vi "hla_incoming_queue_instance_5.vi"(4 "timeout in ms (-1)":i32, 5 "error in (no error)":errorcluster) -> (16 "entity_array":T1[](array[typedef]), 17 "time_step":dbl, 18 "end_simulation":bool, 19 "error out":errorcluster)   [LabVIEW 2016]
uses:
  objects_and_interfaces/InteractionRoot.C2WInteractionRoot.FederateJoinInteraction.ctl
  utilities/runtime/support/controls/queue_assistant_actions.ctl
  utilities/runtime/support/controls/event_assistant_actions.ctl
  utilities/pre-build/support/base_components/controls/incoming_queue_action.ctl
panel:
  out "InteractionRoot.C2WInteractionRoot.FederateJoinInteraction":T1
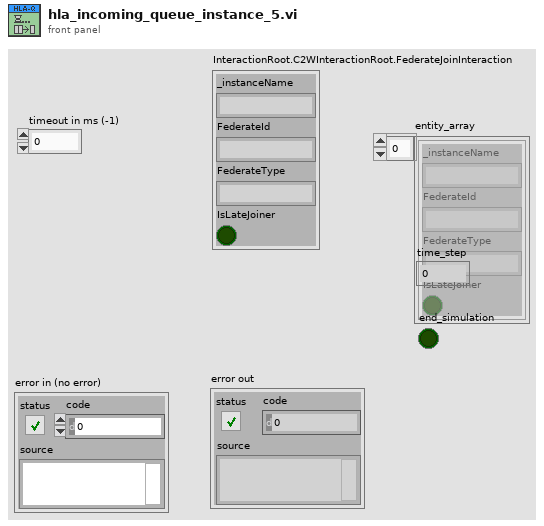
[diagram p1: front panel]
types:
  T1 = typedef "InteractionRoot.C2WInteractionRoot.FederateJoinInteraction.ctl" = cluster{"_instanceName":string, "FederateId":string, "FederateType":string, "IsLateJoiner":bool}
  T2 = typedef "incoming_queue_action.ctl" = enum16{"exit", "process_queue", "wait_on_action"}
  T3 = typedef "event_assistant_actions.ctl" = enum16{"--- unused ---", "destroy", "fire", "get_ref", "init"}
  T4 = typedef "queue_assistant_actions.ctl" = enum16{"--- unused ---", "bulk_enq_ahead", "bulk_enq_behind", "destroy", "empty?", "enq_ahead", "enq_behind", "flush", "get_queues", "init"}
  T5 = typedef "queue_references.ctl" = cluster{"entities_in":refnum<queue>, "entities_out":refnum<queue>, "timestep":refnum<queue>, "response":refnum<queue>}
  T6 = typedef "entity.ctl" = cluster{"type":T7, "classPath":string, "params":string[][], "instanceName":string}
  T7 = typedef "entity_type.ctl" = string
  T8 = typedef "user_events.ctl" = enum16{"abort", "do-step", "sim-end"}
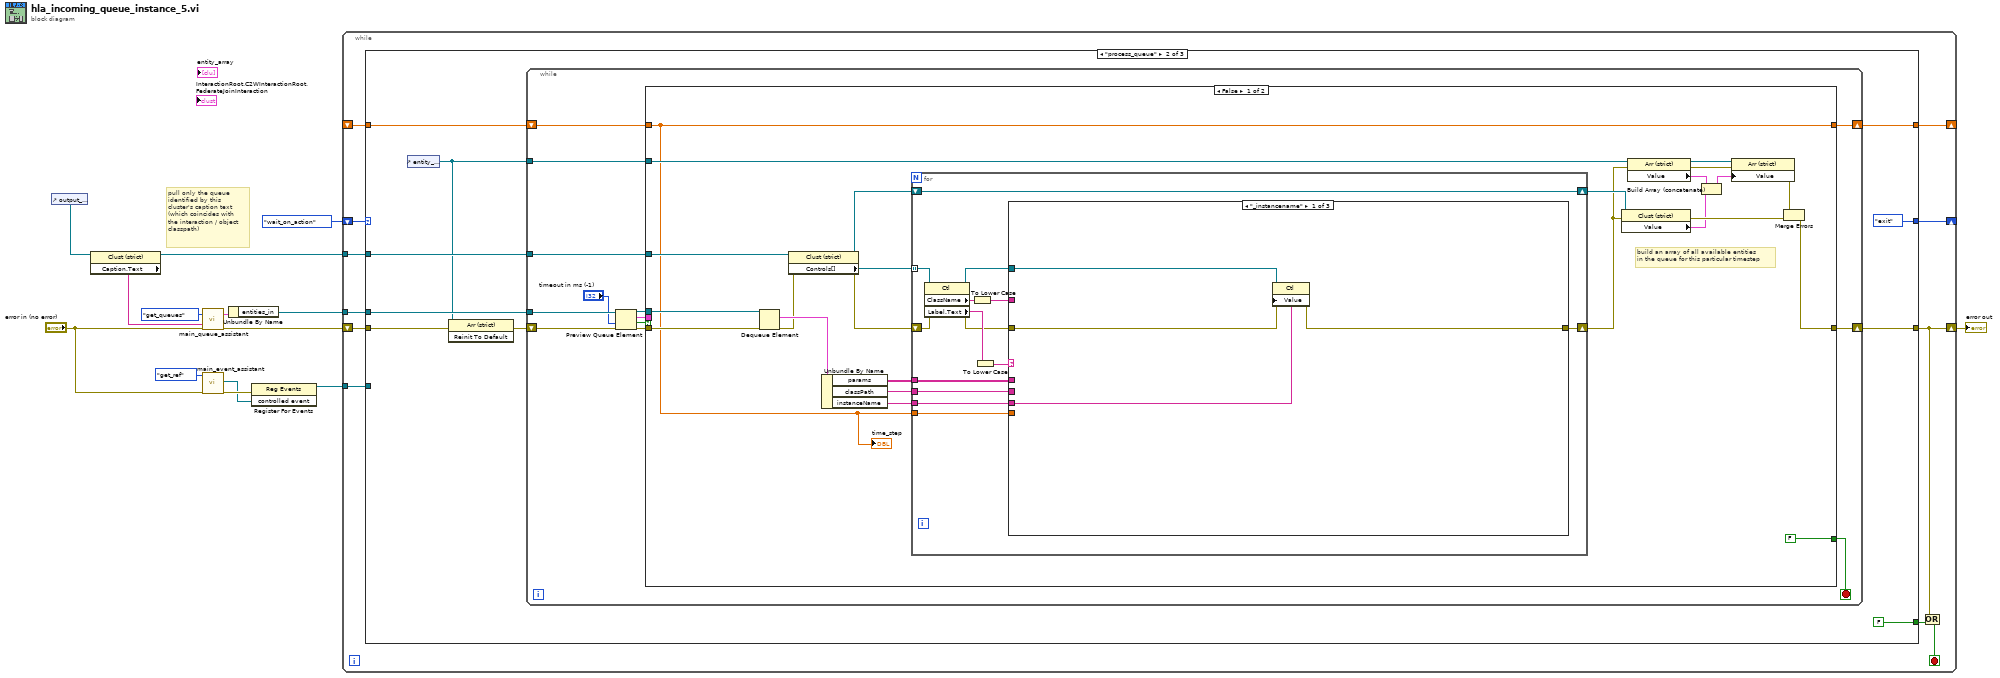
[diagram p0: block diagram]
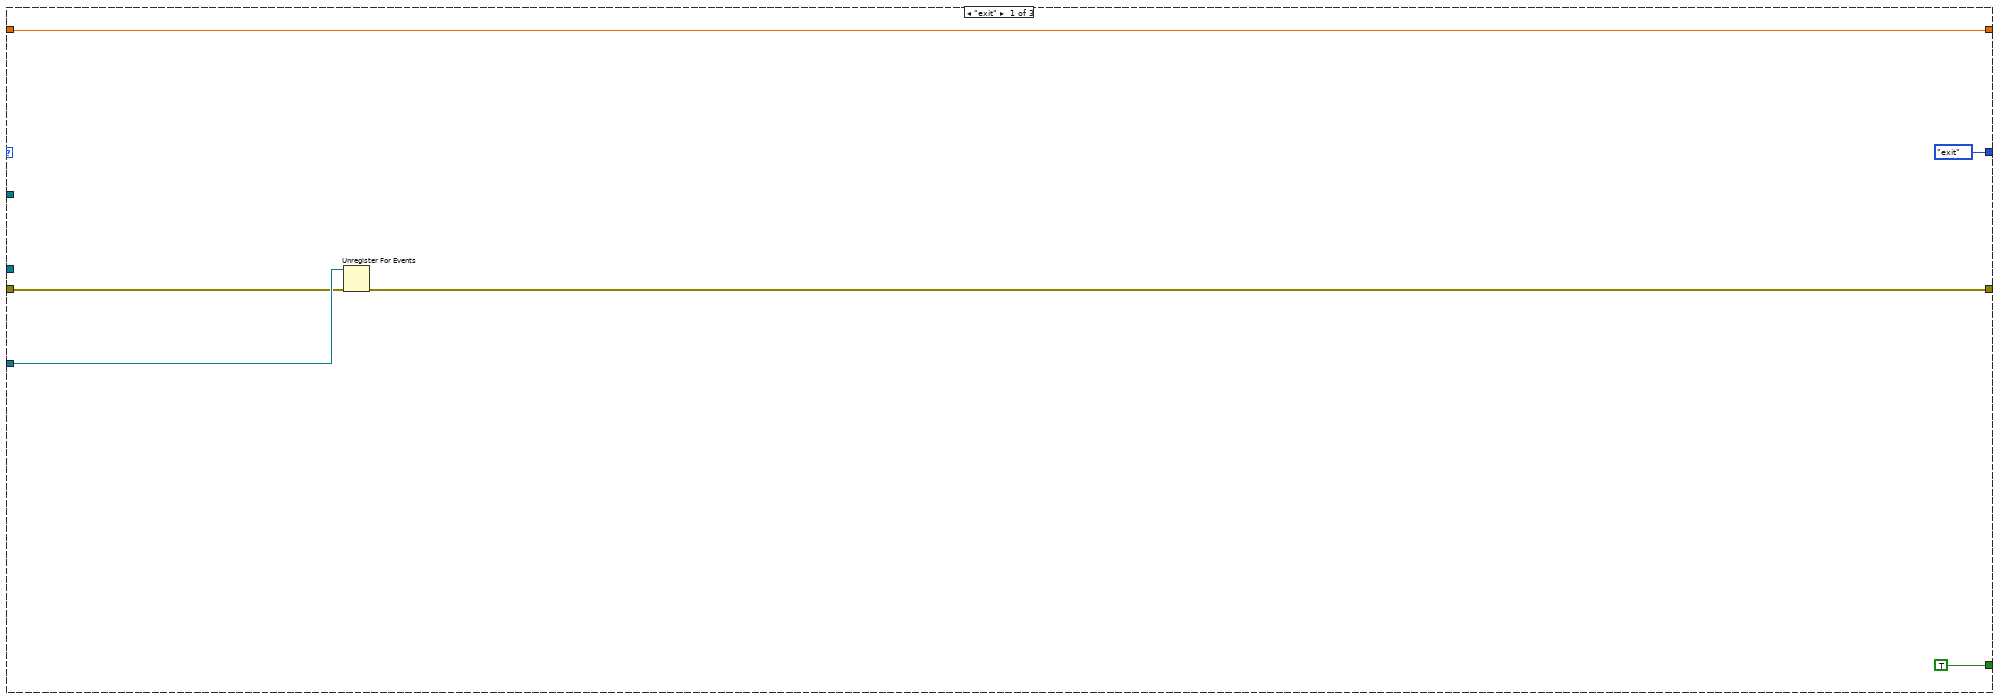
[diagram p2: hidden frame]
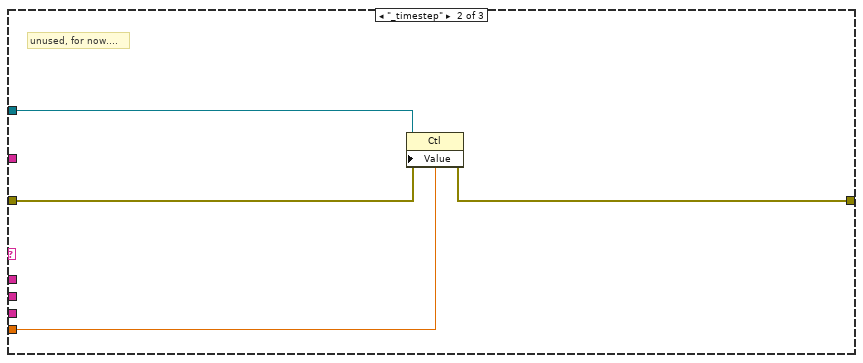
[diagram p3: hidden frame]
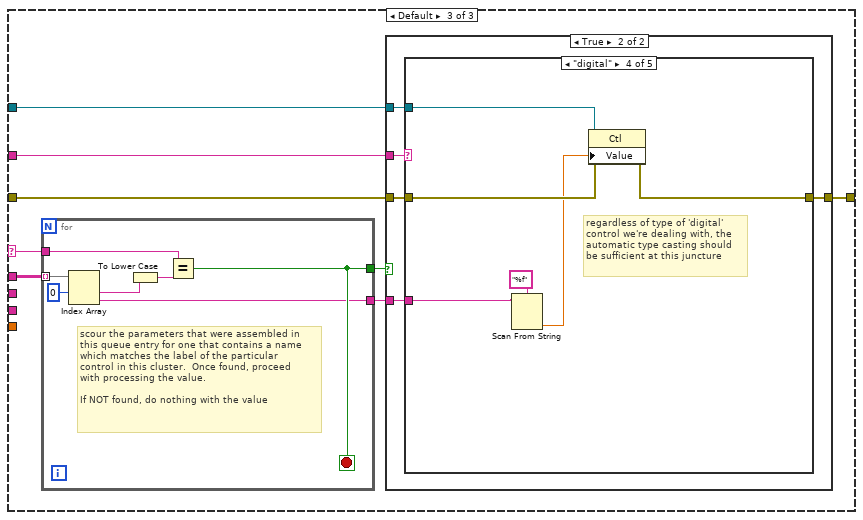
[diagram p4: hidden frame]
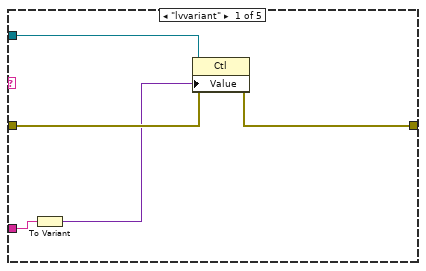
[diagram p6: hidden frame]
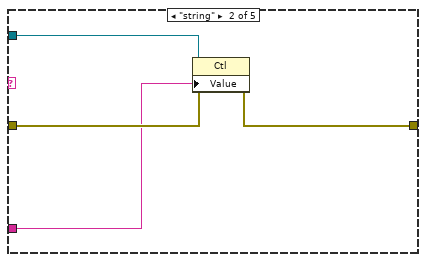
[diagram p7: hidden frame]
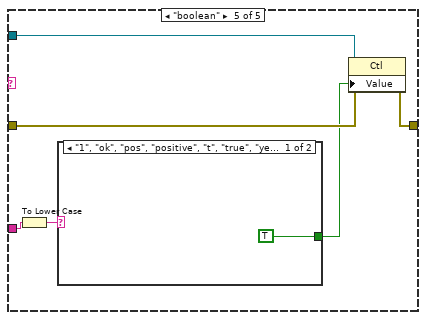
[diagram p9: hidden frame]
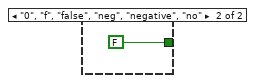
[diagram p10: hidden frame]
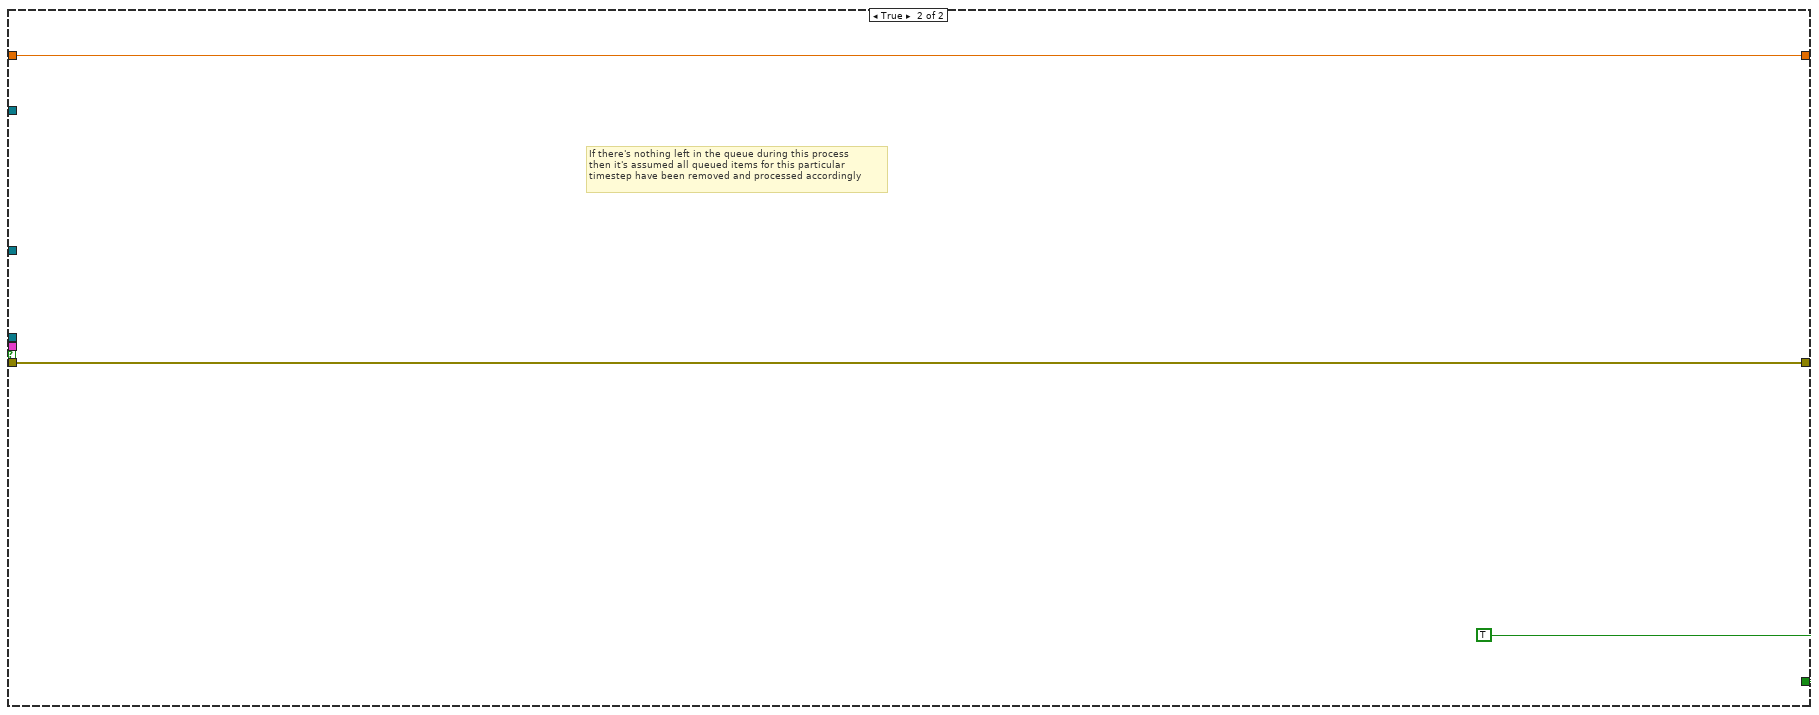
[diagram p11: hidden frame]
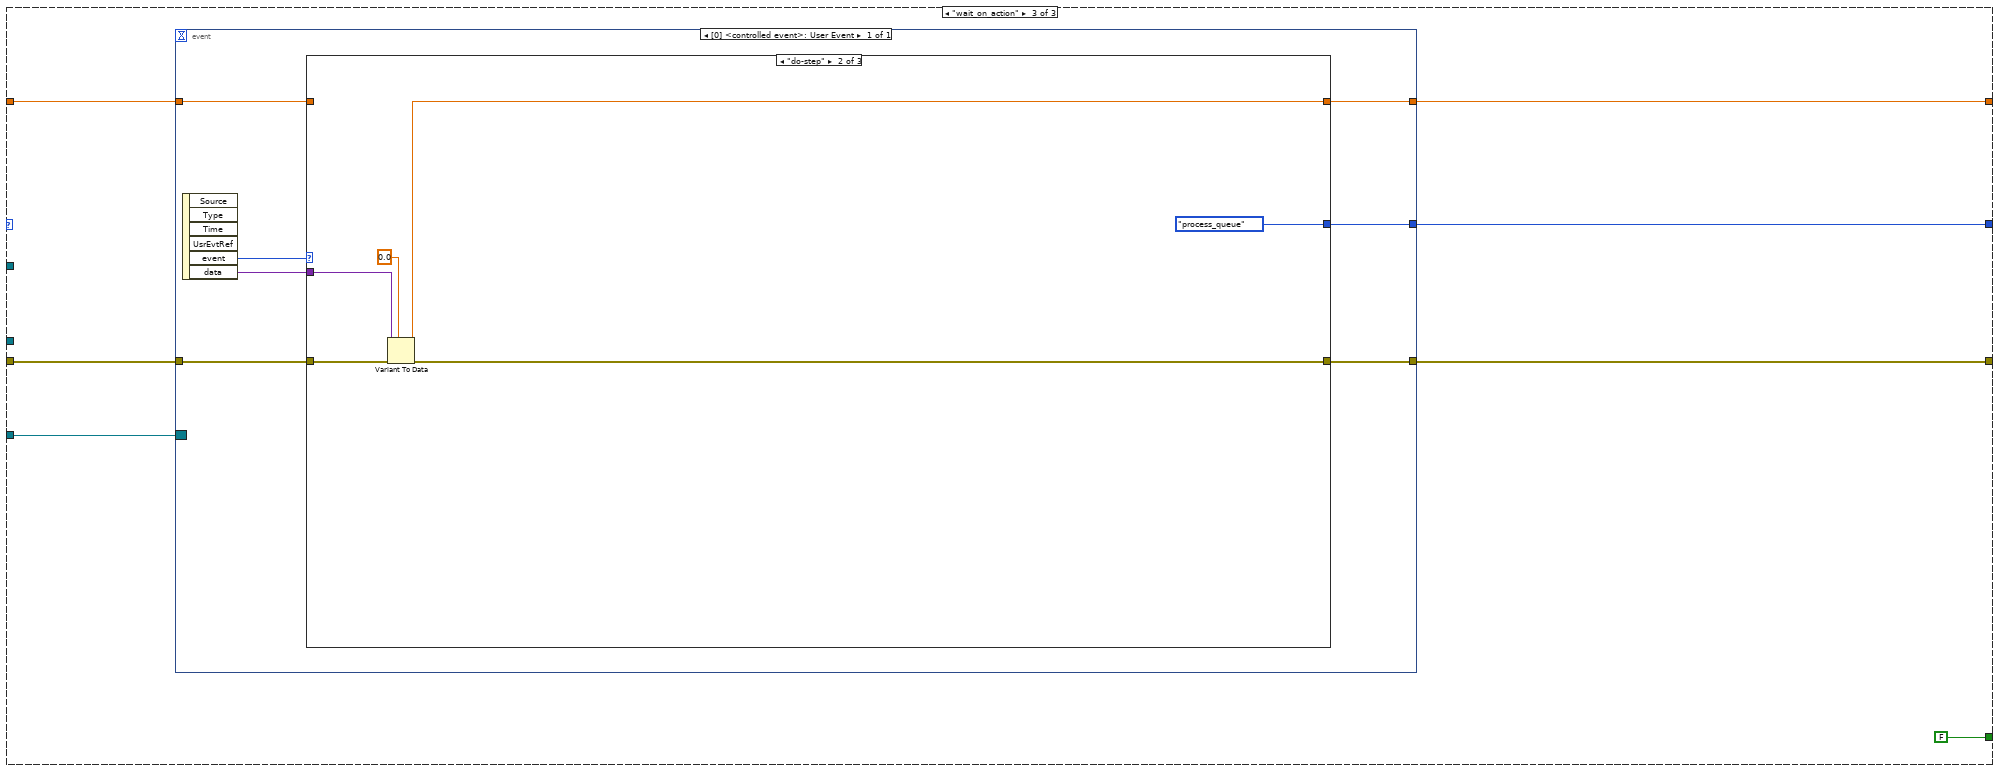
[diagram p12: hidden frame]
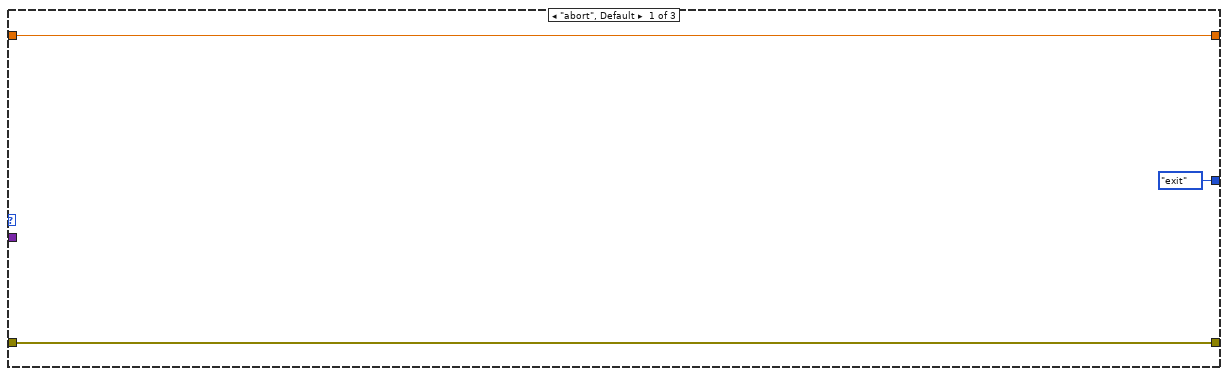
[diagram p13: hidden frame]
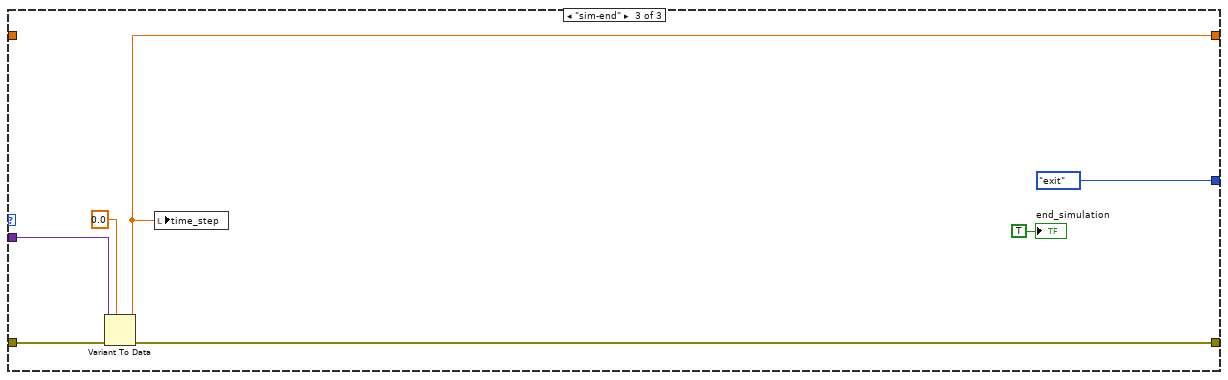
[diagram p14: hidden frame]
diagram:
  # "pull only the queue \nidentified by this \ncluster's caption text\n(which coincides with\nthe interaction / object\nclasspath)"
  n1 = control-ref of="output_cluster"() -> (w3:refnum<vi>)
  n2 = property class="Clust (strict)"(reference=w3) -> (reference out=w11:refnum<vi>, "Caption.Text"=w12:string)  [unwired: 1 in, 1 out]
  n3 = call "main_queue_assistant.vi"("action (enq_behind = def)"=queue_assistant_actions."get_queues" ("queue_action (enq_behind = def)"), "classpath / id (in)"=w12, "error in (no error)"="error in (no error)") -> ("refs (out)"=w2:T5, "error out"=w10:errorcluster)  [unwired: 14 in, 1 out]
  n4 = call "main_event_assistant.vi"("event_action (enq_behind = def)"=event_assistant_actions."get_ref", "error in (no error)"="error in (no error)") -> ("controlled event"=w6:refnum<user-event>, "error out"=w7:errorcluster)  [unwired: 16 in]
  n5 = Unbundle By Name(w2) -> ("entities_in"=w1:refnum<queue>)
  n6 = register-events(error in=w7, w6) -> (reference out=w4:refnum<event-registration>)  [unwired: 1 in, 1 out]
  n7 = while {
    tunnel: w1 -> [w25]
    tunnel: w11 -> [w24]
    shift-right: [w16] -> w13
    shift-left: w10 -> [w23]
    shift-right: [w19] -> _
    shift-left: incoming_queue_action."wait_on_action" -> [w22]
    tunnel: w4 -> [w21]
    shift-right: [w20] -> _
    shift-left: _ -> [w18]
    stop <- w15 stop-if-true
    n8 = case shown="\"process_queue\"" w22 {
      tunnel: w25 -> [_ w41 _]
      tunnel: [w26 w40 w152] -> w16
      tunnel: w24 -> [_ w39 _]
      tunnel: w23 -> [w27 w35 w154]
      tunnel: w21 -> [w28 _ w155]
      tunnel: [w31 w37 w153] -> w20
      tunnel: [incoming_queue_action."exit" incoming_queue_action."exit" w151] -> w19
      tunnel: w18 -> [w31 w36 w150]
      tunnel: [TRUE FALSE FALSE] -> w17
      frame "exit" {
        n9 = Unregister For Events(event registration refnum=w28, error in=w27) -> (error out=w26:errorcluster)
      }
      frame "process_queue" {
        n10 = control-ref of="entity_array"() -> (w33:refnum<vi>)
        n11 = invoke class="Arr (strict)" method="Reinit To Default"(reference=w33, error in=w35) -> (error out=w34:errorcluster)  [unwired: 1 in, 2 out]
        n12 = while {
          tunnel: w41 -> [w54]
          tunnel: w39 -> [w48]
          shift-right: [w49] -> w40
          shift-left: w34 -> [w47]
          shift-right: [w46] -> w37
          shift-left: w36 -> [w45]
          tunnel: w33 -> [w42]
          stop <- w43 stop-if-true
          n13 = Preview Queue Element(queue=w54, timeout in ms (-1)="timeout in ms (-1)", error in (no error)=w47) -> (queue out=w50:refnum<queue>, element=w44:T6, timed out?=w52:bool, error out=w51:errorcluster)
          n14 = case shown="False" w52 {
            tunnel: w51 -> [w75 w148]
            tunnel: w50 -> [w78 _]
            tunnel: [w77 w148] -> w49
            tunnel: w48 -> [w76 _]
            tunnel: w45 -> [w56 w147]
            tunnel: [w56 w147] -> w46
            tunnel: w44 -> [_ _]
            tunnel: [FALSE TRUE] -> w43
            tunnel: w42 -> [w74 _]
            frame False {
              # "build an array of all available entities\nin the queue for this particular timestep"
              n15 = Dequeue Element(queue=w78, error in (no error)=w75) -> (element=w72:T6, error out=w71:errorcluster)  [unwired: 1 in, 2 out]
              n16 = property class="Clust (strict)"(reference=w76, error in=w71) -> (reference out=w62:refnum<vi>, error out=w69:errorcluster, "Controls[]"=w70:refnum<vi>[])
              n17 = Unbundle By Name(w72) -> ("params"=w68:string[][], "classPath"=w67:string, "instanceName"=w55:string)
              n18 = for {
                tunnel: w70 -> [w91] mode=indexing
                tunnel: w68 -> [w87]
                shift-right: [w84] -> w58
                shift-left: w69 -> [w92]
                tunnel: w67 -> [w82]
                shift-right: [w81] -> w61
                shift-left: w62 -> [w81]
                tunnel: w56 -> [w80]
                tunnel: w55 -> [w79]
                n19 = property class="Ctl"(reference=w91, error in=w92) -> (reference out=w89:refnum<vi>, error out=w85:errorcluster, "ClassName"=w90:string, "Label.Text"=w86:string)
                n20 = To Lower Case(string=w90) -> (all lower case string=w88:string)
                n21 = To Lower Case(string=w86) -> (all lower case string=w83:string)
                n22 = case shown="\"_instancename\"" w83 {
                  selector: w83 -> [_ _ w101]
                  tunnel: w89 -> [w96 w100 w108]
                  tunnel: w88 -> [_ _ w107]
                  tunnel: w87 -> [_ _ w106]
                  tunnel: w85 -> [w95 w99 w103]
                  tunnel: [w94 w98 w102] -> w84
                  tunnel: w82 -> [_ _ _]
                  tunnel: w80 -> [_ w97 _]
                  tunnel: w79 -> [w93 _ _]
                  frame "_instancename" {
                    n23 = property class="Ctl"(reference=w96, error in=w95, "Value"=w93) -> (error out=w94:errorcluster)  [unwired: 1 out]
                  }
                  frame "_timestep" {
                    # "unused, for now...."
                    n24 = property class="Ctl"(reference=w100, error in=w99, "Value"=w97) -> (error out=w98:errorcluster)  [unwired: 1 out]
                  }
                  frame Default {
                    n25 = for {
                      tunnel: w106 -> [w142] mode=indexing
                      tunnel: w101 -> [w145]
                      tunnel: [w139] -> w104
                      tunnel: [w143] -> w105
                      stop <- w143 stop-if-true
                      # "scour the parameters that were assembled in\nthis queue entry for one that contains a name\nwhich matches the label of the particular\ncontrol in this cluster.  Once found, proceed\nwith processing the value.\n\nIf NOT found, do nothing with the value"
                      n26 = Index Array(array=w142, index #1=0 ("index")) -> (element #1=w140:string, element #2=w139:string)  [unwired: 1 in]
                      n27 = To Lower Case(string=w140) -> (all lower case string=w144:string)
                      n28 = Equal?(x=w145, y=w144) -> (x = y?=w143:bool)
                    }
                    n29 = case shown="True" w105 {
                      tunnel: w108 -> [_ w114]
                      tunnel: w107 -> [_ w113]
                      tunnel: w104 -> [_ w112]
                      tunnel: w103 -> [w109 w111]
                      tunnel: [w109 w110] -> w102
                      frame False {
                        # "NOT FOUND, disregard this entry"
                      }
                      frame True {
                        n30 = case shown="\"digital\"" w113 {
                          tunnel: w114 -> [w119 w123 _ w130 w136]
                          tunnel: w112 -> [w117 w120 _ w126 w133]
                          tunnel: w111 -> [w118 w122 w124 w129 w135]
                          tunnel: [w115 w121 w124 w128 w134] -> w110
                          frame "lvvariant" {
                            n31 = To Variant(anything=w117) -> (Variant=w116:variant)
                            n32 = property class="Ctl"(reference=w119, error in=w118, "Value"=w116) -> (error out=w115:errorcluster)  [unwired: 1 out]
                          }
                          frame "string" {
                            n33 = property class="Ctl"(reference=w123, error in=w122, "Value"=w120) -> (error out=w121:errorcluster)  [unwired: 1 out]
                          }
                          frame Default {
                            # "if the ClassName is undefined"
                          }
                          frame "digital" {
                            # "regardless of type of 'digital'\ncontrol we're dealing with, the\nautomatic type casting should\nbe sufficient at this juncture"
                            n34 = Scan From String(format string="%f", input string=w126) -> (output 1=w125:dbl)  [unwired: 3 in, 3 out]
                            n35 = property class="Ctl"(reference=w130, error in=w129, "Value"=w125) -> (error out=w128:errorcluster)  [unwired: 1 out]
                          }
                          frame "boolean" {
                            n36 = To Lower Case(string=w133) -> (all lower case string=w132:string)
                            n37 = case shown="\"1\", \"ok\", \"pos\", \"positive\", \"t\", \"true\", \"yes\", Default" w132 {
                              tunnel: [TRUE FALSE] -> w131
                              frame "1", "ok", "pos", "positive", "t", "true", "yes", Default {
                              }
                              frame "0", "f", "false", "neg", "negative", "no" {
                              }
                            }
                            n38 = property class="Ctl"(reference=w136, error in=w135, "Value"=w131) -> (error out=w134:errorcluster)  [unwired: 1 out]
                          }
                        }
                      }
                    }
                  }
                }
              }
              n39 = property class="Clust (strict)"(reference=w61, error in=w58) -> (error out=w59:errorcluster, "Value"=w57:T1)  [unwired: 1 out]
              n40 = property class="Arr (strict)"(reference=w74, error in=w58) -> (reference out=w64:refnum<vi>, error out=w63:errorcluster, "Value"=w66:T1[])
              n41 = Build Array (concatenate)(w66, w57) -> (w65:T1[])
              n42 = property class="Arr (strict)"(reference=w64, error in=w63, "Value"=w65) -> (error out=w60:errorcluster)  [unwired: 1 out]
              n43 = Merge Errors(w60, w59) -> (w77:errorcluster)
              "time_step" <- w56
            }
            frame True {
              # "If there's nothing left in the queue during this process\nthen it's assumed all queued items for this particular\ntimestep have been removed and processed accordingly"
            }
          }
        }
      }
      frame "wait_on_action" {
        n44 = event shown="[0] <controlled event>: User Event" {
          selector: w155 -> [_]
          dyn-events: _ -> [_]
          timeout: _ -> [_]
          tunnel: w154 -> [w160]
          tunnel: [w159] -> w153
          tunnel: [w158] -> w152
          tunnel: [w157] -> w151
          tunnel: w150 -> [w156]
          event User Event {
            n45 = event-data() -> ("event"=w162:T8, "data"=w161:variant)  [unwired: 1 in, 4 out]
            n46 = case shown="\"do-step\"" w162 {
              tunnel: w161 -> [_ w170 w177]
              tunnel: w160 -> [w163 w171 w178]
              tunnel: [w164 w168 w172] -> w159
              tunnel: [w163 w166 w174] -> w158
              tunnel: [incoming_queue_action."exit" incoming_queue_action."process_queue" incoming_queue_action."exit"] -> w157
              tunnel: w156 -> [w164 _ _]
              frame "abort", Default {
              }
              frame "do-step" {
                n47 = Variant To Data(error in=w171, type=0.0, Variant=w170) -> (data=w168:dbl, error out=w166:errorcluster)
              }
              frame "sim-end" {
                n48 = Variant To Data(error in=w178, type=0.0, Variant=w177) -> (data=w172:dbl, error out=w174:errorcluster)
                n49 = local write "time_step"(w172) -> ()
                "end_simulation" <- TRUE ("end_simulation")
              }
            }
          }
        }
      }
    }
    n50 = Or(x=w16, y=w17) -> (x .or. y?=w15:bool)
  }
  "error out" <- w13
